vi "ecg_item_1_to_7.vi"() -> ()   [LabVIEW 2019]
uses:
  <vilib>/Utility/file.llb/Read Delimited Spreadsheet (DBL).vi
  <vilib>/Utility/file.llb/Read Delimited Spreadsheet (string).vi
  <vilib>/measure/NI_MAPro.lvlib
  <vilib>/Analysis/NI_AALPro.lvlib
  <vilib>/express/express analysis/Spectral/XNode/ExpressSpectralMeasurementsBlockNode.xnode
  <vilib>/Analysis/2dsp.llb/Real FFT.vi
  <vilib>/Waveform/WDTOps.llb/WDT Get Waveform Subset DBL.vi
  <vilib>/Analysis/NI_AALBase.lvlib
  <vilib>/Analysis/baseanly.llb/Mean (DBL).vi
  <vilib>/measure/mamon.llb/Waveform Peak Detection for 1 Chan.vi
  <vilib>/express/express analysis/Spectral/Block/exnSpectralBlock spectral measurements power poly.vi
  <vilib>/express/express analysis/Spectral/Block/exnSpectralBlock spectral measurements power WFM.vi
panel:
  in  "Peak detection threshold":dbl format="%.2p"
  out "Total Power":dbl
  in  "Peaks/Valleys":u16(ring) items=["Peaks", "Valleys"]
  in  "Lower Cut-Off freq.":dbl=0.3 caption="Lower Cut-Off"
  in  "Upper Cut-Off freq.":dbl=40.0 caption="Upper Cut-Off"
  out "df":dbl
  out "RR mean":dbl format="%0.2f"
  out "error out":errorcluster
  out "Power Spectrum Magnitude":dbl[](array[numeric])
  out "LF/HF":dbl
  out "HF":dbl
  out "Integral of HF":dynamicdata(graph)
  out "LF":dbl
  out "Integral of LF":dynamicdata(graph)
  out "Integral of TF":dynamicdata(graph)
  out "Power Spectrum":cluster{"f0":dbl, "df":dbl, "magnitude":dbl[]}(graph)
  out "Im{FFT} Graph":dbl[](graph)
  out "Re{FFT} Graph":dbl[](graph)
  out "FFT {X}":cdb[](array[numeric])
  out "RRI FFT magnitude Graph":dbl[](graph)
  out "RRI series":dbl[](graph)
  out "RRI series size":i32
  out "RR interval":dbl[](array[numeric])
  out "peaks found":i32
  out "Band Pass Filter Graph":dynamicdata(graph)
  out "Raw Data Graph":waveform(dbl)(graph)
  in  "file path (dialog if empty)":path
  # "ITEM 1"
  # "ITEM 2"
  # "ITEM 3"
  # "ITEM 4"
  # "ITEM 5"
  # "ITEM 6"
  # "ITEM 7"
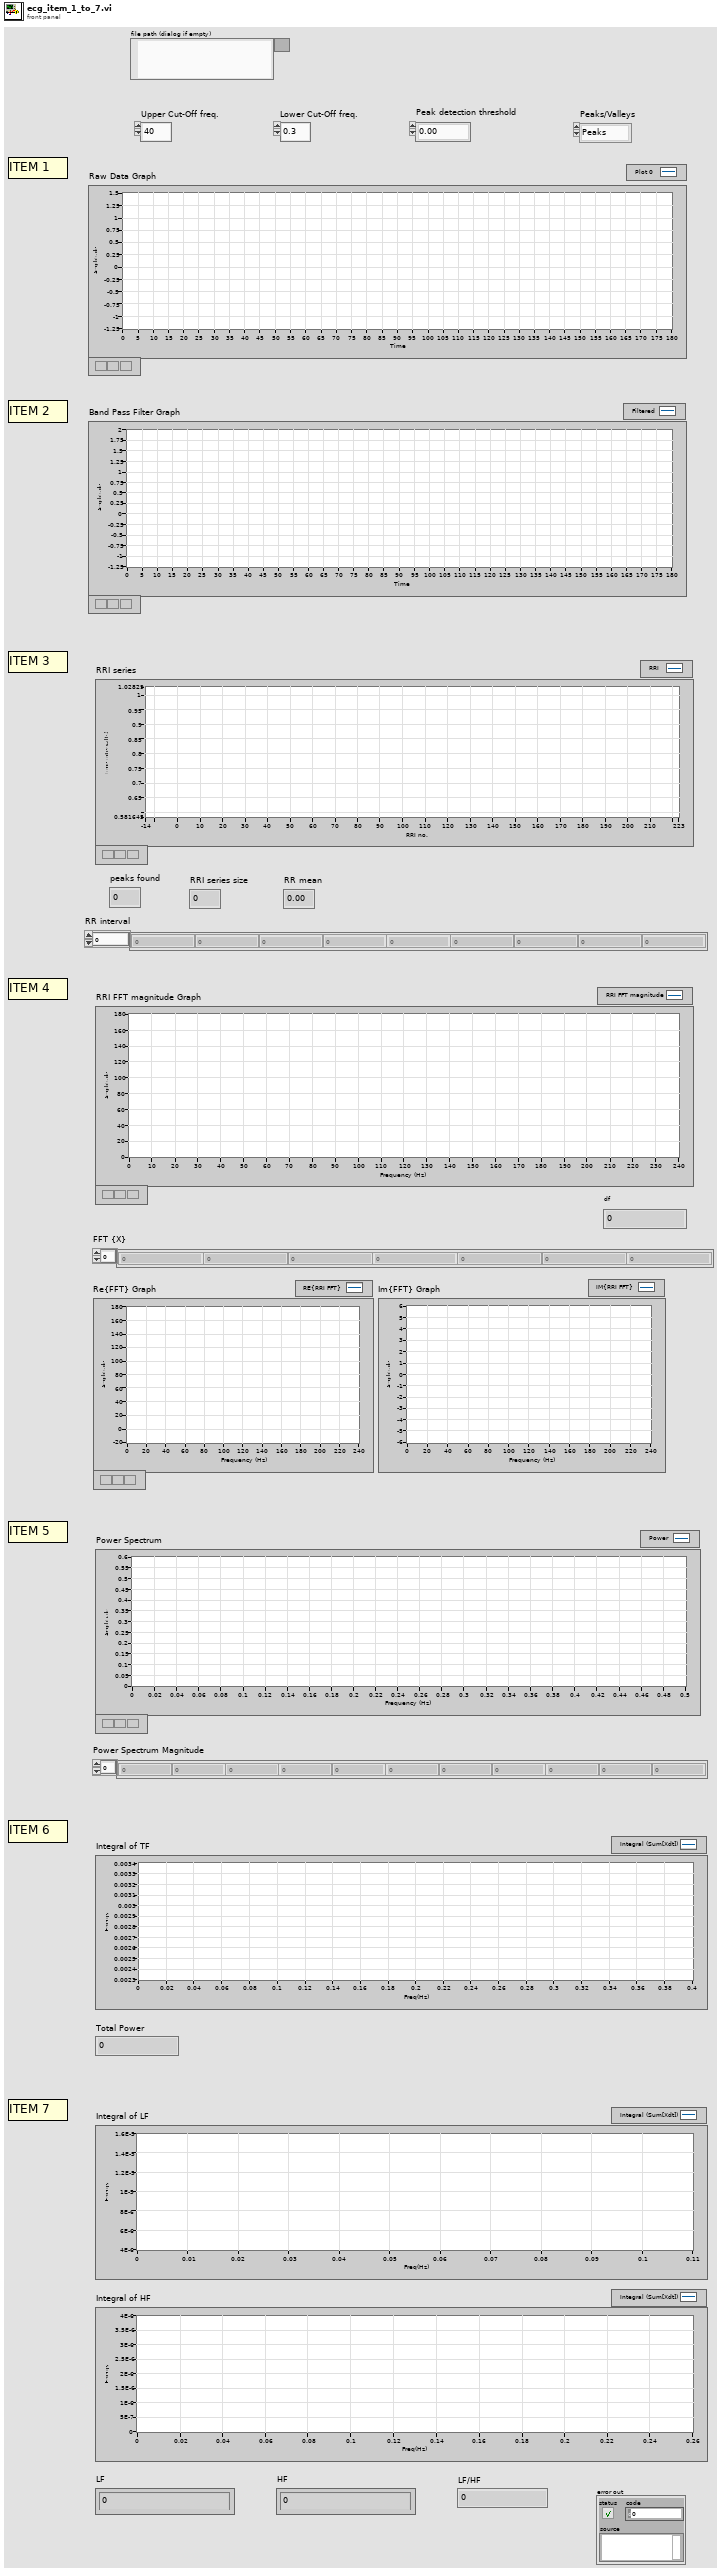
[diagram p1: front panel]
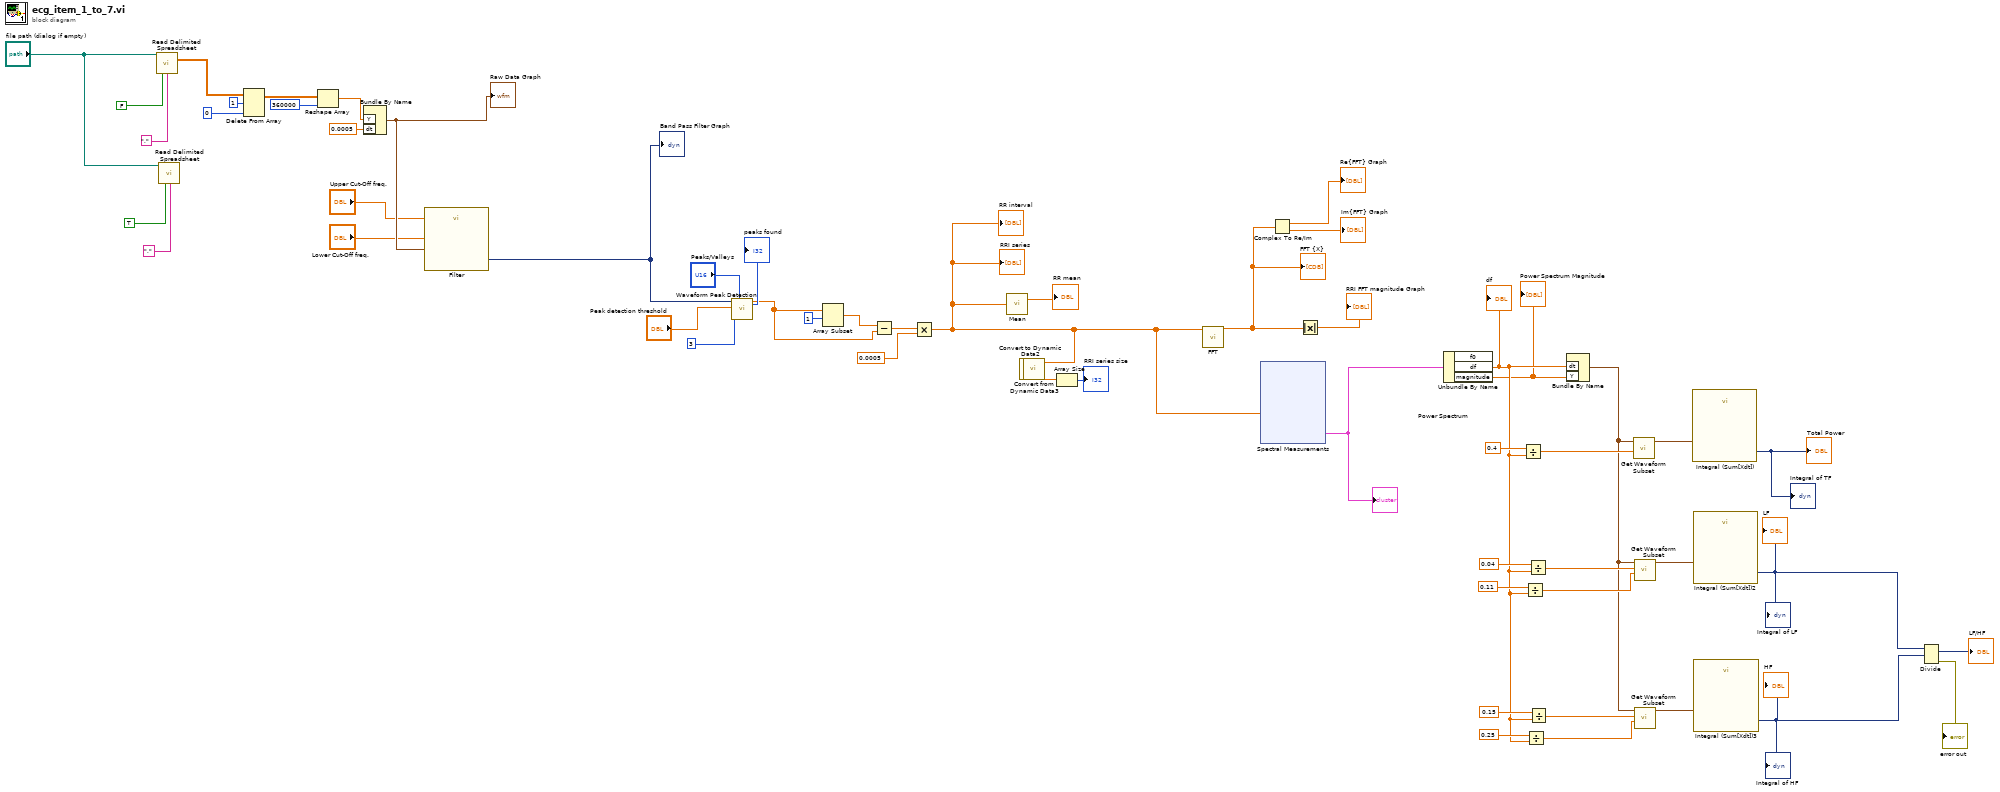
[diagram p0: block diagram]
diagram:
  n1 = call-poly <vilib>:"Read Delimited Spreadsheet.vi"("file path (dialog if empty)"="file path (dialog if empty)", "transpose? (F)"=FALSE, "delimiter (\\t)"="," ("delimiter (\\t)")) -> ("all rows"=w49:dbl[][])  [unwired: 7 in, 5 out]
  n2 = call-poly <vilib>:"Read Delimited Spreadsheet.vi"("file path (dialog if empty)"="file path (dialog if empty)", "transpose? (F)"=TRUE, "delimiter (\\t)"="," ("delimiter (\\t)")) -> ()  [unwired: 7 in, 6 out]
  n3 = Delete From Array(array=w49, length=1, index (col)=0 ("disabled index (col)")) -> (array with subset deleted=w48:dbl[][])  [unwired: 1 in, 1 out]
  n4 = Reshape Array(w48, 360000 ("dimension size")) -> (w41:dbl[])
  n5 = Bundle By Name("Y"=w41, "dt"=0.0005) -> (w13:waveform(dbl))  [unwired: 1 in]
  "Raw Data Graph" <- w13
  n6 = call "Filter"("Lower Cut-Off"="Lower Cut-Off freq.", "Upper Cut-Off"="Upper Cut-Off freq.", "Signal"=w13) -> ("Filtered Signal"=w11:dynamicdata)  [unwired: 7 in, 1 out]
  "Band Pass Filter Graph" <- w11
  n7 = call-poly <vilib>:"Waveform Peak Detection.vi"("peaks/valleys"="Peaks/Valleys", "width"=3, "threshold"="Peak detection threshold", "Signal In"=w11) -> ("Locations"=w43:dbl[], "# found"=→"peaks found":i32)  [unwired: 3 in, 3 out]
  n8 = Array Subset(array=w43, index=1) -> (w42:dbl[])  [unwired: 1 in]
  n9 = Subtract(x=w42, y=w43) -> (x-y=w30:dbl[])
  n10 = Multiply(x=w30, y=0.0005) -> (x*y=w10:dbl[])
  "RR interval" <- w10
  "RRI series" <- w10
  n11 = call-poly <vilib>:"Mean.vi"("X"=w10) -> ("mean"=→"RR mean":dbl)  [unwired: 1 out]
  n12 = call "Convert to Dynamic Data2"("Array"=w10) -> ("Dynamic Data Type"=w31:dynamicdata)  [unwired: 3 in]
  n13 = call "Convert from Dynamic Data3"("Dynamic Data Type"=w31) -> ("Array"=w36:dbl[])  [unwired: 3 in]
  n14 = Array Size(array=w36) -> (size(s)=→"RRI series size":i32)
  n15 = call-poly <vilib>:"FFT.vi"("X"=w10) -> ("FFT {X}"=w9:cdb[])  [unwired: 9 in, 1 out]
  "FFT {X}" <- w9
  n16 = xnode "Spectral Measurements"("Signals"=w10) -> ("Power Spectrum"=w8:cluster{"f0":dbl, "df":dbl, "magnitude":dbl[]})  [unwired: 1 in, 1 out]
  "Power Spectrum" <- w8
  n17 = Complex To Re/Im(x + iy=w9) -> (x=→"Re{FFT} Graph":dbl[], y=→"Im{FFT} Graph":dbl[])
  n18 = Absolute Value(x=w9) -> (abs(x)=→"RRI FFT magnitude Graph":dbl[])
  n19 = Unbundle By Name(w8) -> ("df"=w7:dbl, "magnitude"=w6:dbl[])  [unwired: 1 out]
  "Power Spectrum Magnitude" <- w6
  "df" <- w7
  n20 = Divide(x=0.4, y=w7) -> (x/y=w33:dbl)
  n21 = Divide(x=0.11, y=w7) -> (x/y=w26:dbl)
  n22 = Divide(x=0.25, y=w7) -> (x/y=w21:dbl)
  n23 = Divide(x=0.04, y=w7) -> (x/y=w25:dbl)
  n24 = Divide(x=0.15, y=w7) -> (x/y=w22:dbl)
  n25 = Bundle By Name("dt"=w7, "Y"=w6) -> (w18:waveform(dbl))  [unwired: 1 in]
  n26 = call-poly <vilib>:"Get Waveform Subset.vi"("duration"=w33, "waveform in"=w18) -> ("waveform out"=w32:waveform(dbl))  [unwired: 4 in, 3 out]
  n27 = call-poly <vilib>:"Get Waveform Subset.vi"("duration"=w26, "start samples/time"=w25, "waveform in"=w18) -> ("waveform out"=w28:waveform(dbl))  [unwired: 3 in, 3 out]
  n28 = call-poly <vilib>:"Get Waveform Subset.vi"("duration"=w21, "start samples/time"=w22, "waveform in"=w18) -> ("waveform out"=w19:waveform(dbl))  [unwired: 3 in, 3 out]
  n29 = call "Integral (Sum[Xdt])"("Signals"=w32) -> ("Result"=→"Integral of TF" →"Total Power":dynamicdata)  [unwired: 5 in, 1 out]
  n30 = call "Integral (Sum[Xdt])2"("Signals"=w28) -> ("Result"=w16:dynamicdata)  [unwired: 5 in, 1 out]
  "LF" <- w16
  "Integral of LF" <- w16
  n31 = call "Integral (Sum[Xdt])3"("Signals"=w19) -> ("Result"=w15:dynamicdata)  [unwired: 5 in, 1 out]
  "HF" <- w15
  "Integral of HF" <- w15
  n32 = Divide(1:w15, 2:w16) -> (0:→"LF/HF":dynamicdata, 3:→"error out":errorcluster)  [unwired: 1 in]
